vi "FRAS Construction tab Y.vi"(5 "Largeur cote":i32, 9 "Tableau":i32[](array[numeric])) -> (8 "Tableau 2":i32[](array[numeric]))   [LabVIEW 2020]
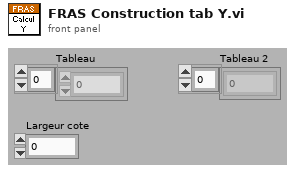
[diagram p1: front panel]
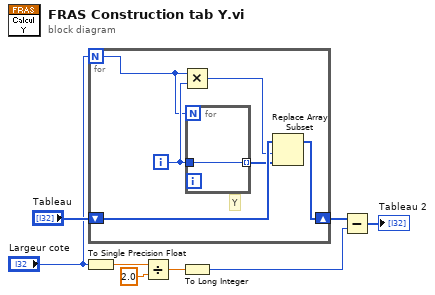
[diagram p0: block diagram]
diagram:
  n1 = To Single Precision Float(number="Largeur cote") -> (single precision float=w1:sgl)
  n2 = for {
    N: "Largeur cote" -> [w9]
    shift-right: [w14] -> w5
    shift-left: "Tableau" -> [w13]
    i -> [w10]
    # "Y"
    n3 = Multiply(x=w9, y=w10) -> (x*y=w12:i32)
    n4 = for {
      N: w9 -> [_]
      tunnel: [w15] -> w11 mode=indexing
      tunnel: w10 -> [w15]
    }
    n5 = Replace Array Subset(array=w13, new element=w11, index=w12) -> (w14:i32[])
  }
  n6 = Divide(x=w1, y=sgl 2.0) -> (x/y=w7:sgl)
  n7 = To Long Integer(number=w7) -> (32bit integer=w6:i32)
  n8 = Subtract(x=w5, y=w6) -> (x-y=→"Tableau 2":i32[])
